vi "Set Scene Item Enabled.vi"(6 "Enabled":bool, 8 "error in (no error)":errorcluster, 9 "Item ID":i32, 10 "Scene Name":string, 11 "OBS in":refnum<class "OBS.lvclass">) -> (0 "error out":errorcluster, 3 "OBS out":refnum<class "OBS.lvclass">)   [LabVIEW 2020, in "obs-websocket.lvlib" / "OBS.lvclass"]
uses:
  OBS.lvclass
  OBS.lvclass/OBS.ctl
  SetSceneItemEnabled/SetSceneItemEnabled.lvclass
  REmptyResponse/REmptyResponse.lvclass
  C:/dev/lv20CE/lv-obs-websocket/obs-websocket-lv/Response/Response.lvclass
  C:/dev/lv20CE/lv-obs-websocket/obs-websocket-lv/Server Message/Server Message.lvclass
  C:/dev/lv20CE/lv-obs-websocket/obs-websocket-lv/Message/Message.lvclass
  C:/dev/lv20CE/lv-obs-websocket/obs-websocket-lv/REmptyResponse/REmptyResponse.lvclass
  C:/dev/lv20CE/lv-obs-websocket/obs-websocket-lv/Request/Request.lvclass
  C:/dev/lv20CE/lv-obs-websocket/obs-websocket-lv/Client Message/Client Message.lvclass
  C:/dev/lv20CE/lv-obs-websocket/obs-websocket-lv/SetSceneItemEnabled/SetSceneItemEnabled.lvclass
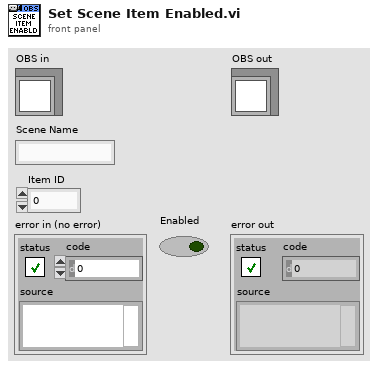
[diagram p1: front panel]
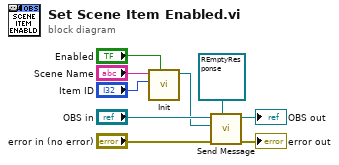
[diagram p0: block diagram]
diagram:
  n1 = call "Init.vi"("Enabled"="Enabled", "Item ID"="Item ID", "Scene Name"="Scene Name") -> ("SetSceneItemEnabled out"=w4:refnum<class "SetSceneItemEnabled.lvclass">)  [unwired: 7 in, 1 out]
  n2 = call "Send Message.vi"("Response Type (None)"=refnum<class "REmptyResponse.lvclass"> refnum ("obs-websocket-lv.lvlib:REmptyResponse.lvclass"), "error in (no error)"="error in (no error)", "Client Message"=w4, "OBS in"="OBS in") -> ("error out"=→"error out":errorcluster, "OBS in"=→"OBS out":refnum<class "OBS.lvclass">)  [unwired: 4 in, 2 out]
